vi "get_publishers.vi"(8 "error in (no error)":errorcluster, 11 "publishers path":path) -> (0 "error out":errorcluster, 3 "publisher map":T1)   [LabVIEW 2024, in "manager_daemon.lvclass"]
uses:
  manager_daemon.lvclass
  type_defs/PublisherMap--map.ctl
  type_defs/PublisherData--cluster.ctl
  CV_Shared_Library/CV_Shared_Library.lvlib
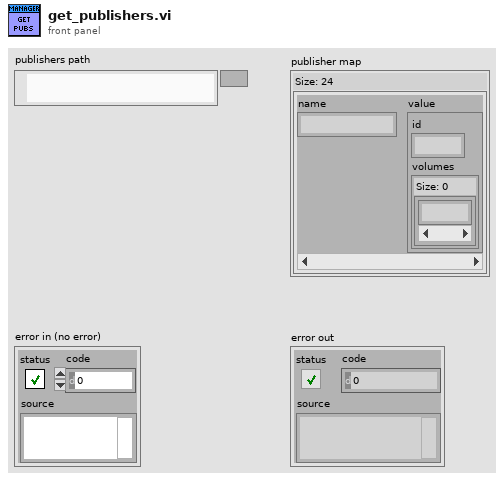
[diagram p1: front panel]
types:
  T1 = typedef "manager_daemon.lvclass/PublisherMap--map.ctl" = map{string, T2}
  T2 = typedef "manager_daemon.lvclass/PublisherData--cluster.ctl" = cluster{"id":i32, "volumes":set{i32}}
  T3 = typedef "CV_RESTful_Lib.lvlib/local_publisher--cluster.ctl" = cluster{"id":i32, "name":string, "sortable_name":string, "aliases":string[], "description":string, "deck":string, "site_detail_url":string, "date_last_updated":timestamp, "cv_id":string, "volume_ids":i32[]}
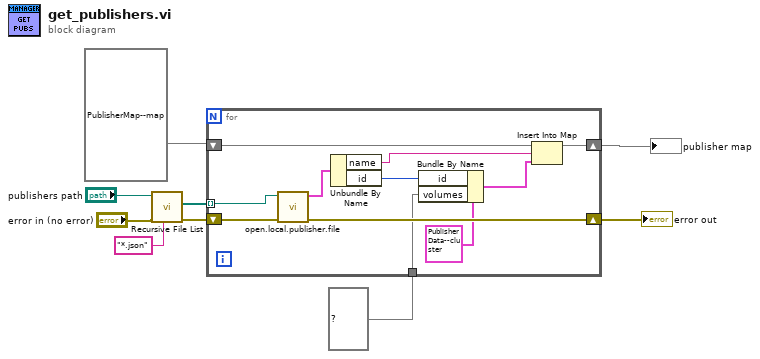
[diagram p0: block diagram]
diagram:
  n1 = call <vilib>:"Recursive File List.vi"("pattern"="*.json", "error in (no error)"="error in (no error)", "Folder Path"="publishers path") -> ("error out"=w7:errorcluster, "All Files in Dir"=w6:path[])  [unwired: 4 in, 3 out]
  n2 = for {
    shift-right: [w18] -> w3
    shift-left: w7 -> [w20]
    tunnel: w6 -> [w19] mode=indexing
    shift-right: [w15] -> w5
    shift-left: T1 {} ("map") -> [w16]
    tunnel: set{i32} {} ("volumes") -> [w11]
    n3 = call "open.local.publisher.file.vi"("error in (no error)"=w20, "publisher json"=w19) -> ("error out"=w18:errorcluster, "publisher"=w17:T3)  [unwired: 8 in]
    n4 = Unbundle By Name(w17) -> ("name"=w14:string, "id"=w12:i32)
    n5 = Bundle By Name(cluster=T2 {"id"=0, "volumes"={}} ("output cluster"), "id"=w12, "volumes"=w11) -> (w10:T2)
    n6 = Insert Into Map(map in=w16, key=w14, value=w10) -> (map out=w15:T1)  [unwired: 2 out]
  }
  "publisher map" <- w5
  "error out" <- w3
